vi "Сумматор 1.vi"(2 "C":bool, 3 "B":bool, 4 "A":bool) -> (0 "S1":bool, 1 "SO":bool)   [LabVIEW 2017]
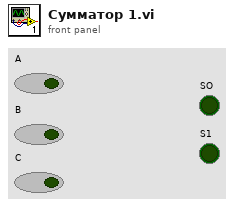
[diagram p1: front panel]
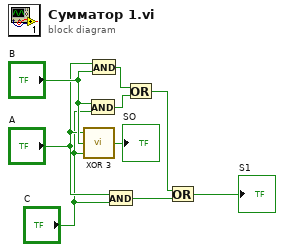
[diagram p0: block diagram]
diagram:
  n1 = call "XOR 3.vi"("z"="C", "y 2"="B", "x"="A") -> ("ok"=→"SO":bool)
  n2 = And(x="B", y="C") -> (x .and. y?=w5:bool)
  n3 = And(x="A", y="B") -> (x .and. y?=w6:bool)
  n4 = And(x="A", y="C") -> (x .and. y?=w3:bool)
  n5 = Or(x=w6, y=w5) -> (x .or. y?=w4:bool)
  n6 = Or(x=w4, y=w3) -> (x .or. y?=→"S1":bool)
